vi "EAGLE Structure 2 Table.vi"(10 "Eagle Data":T1) -> (2 "TableOut":string[][](table)=[["Patient Number", "057235558", ""], ["Eye", "Right Eye", ""], ["Treatment Area", "Full 360", ""], ["Eye Color", "Blue/Green", ""], ["Avg. Pulse Energy", "1.4mJ", ""], ["Number of Pulses", "100", ""], ["Time Between Pulses", "8.0mSec", ""], ["Distance from Limbus", "200.0um", ""], ["Illumination Intensity", "12", ""], ["Aiming Beam Intensity", "5", ""], ["Raneging Beam Intensity", "5", ""]])   [LabVIEW 2015]
uses:
  Controls/Eagle Data.ctl
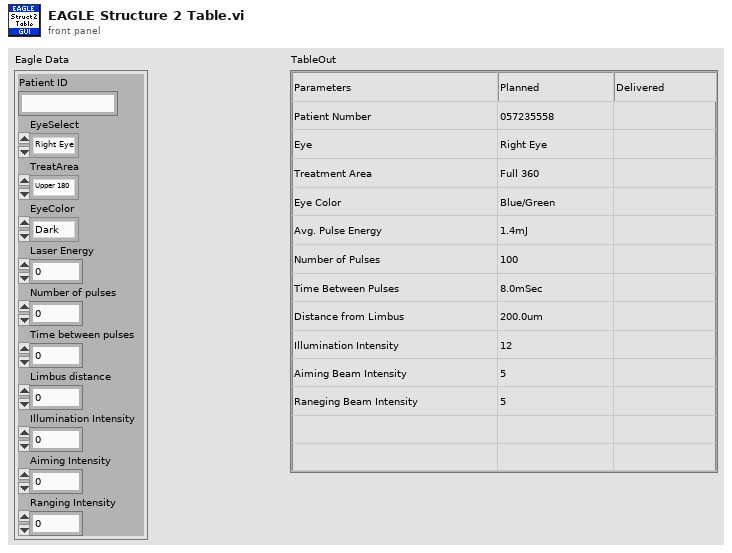
[diagram p1: front panel]
types:
  T1 = typedef "Eagle Data.ctl" = cluster{"Patient ID":string, "EyeSelect":enum32{"Right Eye", "Left Eye"}, "TreatArea":enum32{"Upper 180", "Lower 180", "Full 360"}, "EyeColor":enum32{"Dark", "Bright"}, "Laser Energy":dbl, "Number of pulses":u32, "Time between pulses":dbl, "Limbus distance":dbl, "Illumination Intensity":dbl, "Aiming Intensity":dbl, "Ranging Intensity":dbl}
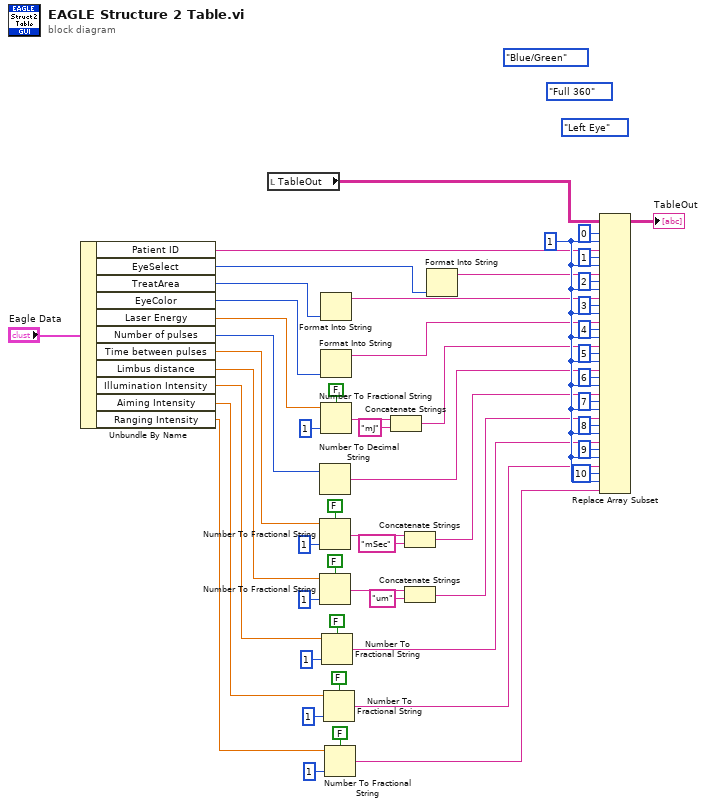
[diagram p0: block diagram]
diagram:
  w51 = 1 ("disabled index (col)")
  (unwired) enum32{"Right Eye", "Left Eye"}."Left Eye" ("EyeSelect")
  (unwired) enum32{"Upper 180", "Lower 180", "Full 360"}."Full 360" ("TreatArea")
  (unwired) enum32{"Dark", "Blue/Green"}."Blue/Green" ("EyeColor")
  n1 = Unbundle By Name("Eagle Data") -> ("Patient ID"=w39:string, "EyeSelect"=w38:enum32{"Right Eye", "Left Eye"}, "TreatArea"=w36:enum32{"Upper 180", "Lower 180", "Full 360"}, "EyeColor"=w34:enum32{"Dark", "Bright"}, "Laser Energy"=w32:dbl, "Number of pulses"=w26:u32, "Time between pulses"=w20:dbl, "Limbus distance"=w14:dbl, "Illumination Intensity"=w10:dbl, "Aiming Intensity"=w6:dbl, "Ranging Intensity"=w2:dbl)
  n2 = local read "TableOut"() -> (w53:string[][])
  n3 = Number To Decimal String(number=w26) -> (decimal integer string=w25:string)  [unwired: 1 in]
  n4 = Number To Fractional String(use system decimal point (T)=FALSE, number=w20, precision (6)=i16 1) -> (F-format string=w22:string)  [unwired: 1 in]
  n5 = Number To Fractional String(use system decimal point (T)=FALSE, number=w14, precision (6)=i16 1) -> (F-format string=w17:string)  [unwired: 1 in]
  n6 = Format Into String(w36) -> (resulting string=w35:string)  [unwired: 3 in, 1 out]
  n7 = Format Into String(w34) -> (resulting string=w33:string)  [unwired: 3 in, 1 out]
  n8 = Number To Fractional String(use system decimal point (T)=FALSE, number=w32, precision (6)=i16 1) -> (F-format string=w30:string)  [unwired: 1 in]
  n9 = Number To Fractional String(use system decimal point (T)=FALSE, number=w10, precision (6)=i16 1) -> (F-format string=w9:string)  [unwired: 1 in]
  n10 = Number To Fractional String(use system decimal point (T)=FALSE, number=w6, precision (6)=i16 1) -> (F-format string=w5:string)  [unwired: 1 in]
  n11 = Number To Fractional String(use system decimal point (T)=FALSE, number=w2, precision (6)=i16 1) -> (F-format string=w1:string)  [unwired: 1 in]
  n12 = Concatenate Strings(w30, "mJ" ("string")) -> (w28:string)
  n13 = Concatenate Strings(w22, "mSec" ("string")) -> (w19:string)
  n14 = Concatenate Strings(w17, "um" ("string")) -> (w13:string)
  n15 = Format Into String(w38) -> (resulting string=w37:string)  [unwired: 3 in, 1 out]
  n16 = Replace Array Subset(array=w53, new element #1=w39, index (row) #1=0 ("disabled index (row)"), index (col) #1=w51, new element #2=w37, index (row) #2=1 ("disabled index (row)"), index (col) #2=w51, new element #3=w35, index (row) #3=2 ("disabled index (row)"), index (col) #3=w51, new element #4=w33, index (row) #4=3 ("disabled index (row)"), index (col) #4=w51, new element #5=w28, index (row) #5=4 ("disabled index (row)"), index (col) #5=w51, new element #6=w25, index (row) #6=5 ("disabled index (row)"), index (col) #6=w51, new element #7=w19, index (row) #7=6 ("disabled index (row)"), index (col) #7=w51, new element #8=w13, index (row) #8=7 ("disabled index (row)"), index (col) #8=w51, new element #9=w9, index (row) #9=8 ("disabled index (row)"), index (col) #9=w51, new element #10=w5, index (row) #10=9 ("disabled index (row)"), index (col) #10=w51, new element #11=w1, index (row) #11=10 ("disabled index (row)"), index (col) #11=w51) -> (→"TableOut":string[][])
